vi "PID Straight Encoder.vi"(8 "error in":errorcluster, 10 "data":variant=variant(dbl -50.0), 11 "Auton Ref":T1={"queue"=refnum, "Drivetrain"={"DevStatus"={"status"=FALSE, "code"=0, "source"=""}, "Motors[]"=[{"DeviceStatus"={"status"=FALSE, "code"=0, "source"=""}, "Type"=enum."PWM", "PWM"={"PWM Channel"=enum."PWM 1", "DeadBand"={"Name"="SPARK", "maxPositivePwm"=1500, "minPositivePwm"=1010, "centerPwm"=1005, "maxNegativePwm"=1000, "minNegativePwm"=500, "angularRange"=0}}, "CAN"={"Device Number"=0, "SetOutput VI Ref"=variant(refnum<vi> refnum), "GetOutput VI Ref"=variant(refnum<vi> refnum), "Enable VI Ref"=variant(refnum<vi> refnum), "Disable VI Ref"=variant(refnum<vi> refnum), "Data"=variant}, "Invert"=TRUE}, {"DeviceStatus"={"status"=FALSE, "code"=0, "source"=""}, "Type"=enum."PWM", "PWM"={"PWM Channel"=enum."PWM 0", "DeadBand"={"Name"="SPARK", "maxPositivePwm"=1500, "minPositivePwm"=1010, "centerPwm"=1005, "maxNegativePwm"=1000, "minNegativePwm"=500, "angularRange"=0}}, "CAN"={"Device Number"=0, "SetOutput VI Ref"=variant(refnum<vi> refnum), "GetOutput VI Ref"=variant(refnum<vi> refnum), "Enable VI Ref"=variant(refnum<vi> refnum), "Disable VI Ref"=variant(refnum<vi> refnum), "Data"=variant}, "Invert"=FALSE}], "Square Inputs"=TRUE, "Max Output"=1.0}, "Encoder L"={"DevStatus"={"status"=FALSE, "code"=0, "source"=""}, "EncoderIndex"=enum."Enc 0", "CounterIndex"=enum."Invalid", "DistancePerCount"=0.0490874, "Decoding Type"=enum."4x"}, "Encoder R"={"DevStatus"={"status"=FALSE, "code"=0, "source"=""}, "EncoderIndex"=enum."Enc 1", "CounterIndex"=enum."Invalid", "DistancePerCount"=0.0490874, "Decoding Type"=enum."4x"}, "Gyro"={"DevStatus"={"status"=FALSE, "code"=0, "source"=""}, "Analog Channel"=enum."AI 1", "Offset"=0.0, "Gain (VoltsPerDegree/Second)"=0.0, "Gyro Type"=enum."XRS450", "Handle"=60, "SPI Bus"=enum."SPI On-Board, CS0", "Device Found"=TRUE, "Sample Rate"=1.0, "Calibrate On Open"=FALSE}, "Lock"={"notifier out"=refnum}, "Shifter"={"DevStatus"={"status"=FALSE, "code"=0, "source"=""}, "Pneumatics Control Module"=1, "Forward Solenoid Channel"=enum."Solenoid 0", "Reverse Solenoid Channel"=enum."Solenoid 1"}} {"Gyro"."Sample Rate" min=0.25 max=100.0 step=0.25}) -> (0 "error out":errorcluster)   [LabVIEW 2016, in "Drive System.lvlib"]
uses:
  Drive System.lvlib
  DriveMainType.ctl
  DriveCmd.ctl
  DriveCmdList.ctl
  <vilib>/Rock Robotics/WPI/RobotDrive/WPI_RobotDriveDevRef.ctl
  <vilib>/Rock Robotics/WPI/MotorControl/WPI_MotorControlDeviceRef.ctl
  <vilib>/Rock Robotics/WPI/MotorControl/WPI_MotorControlType.ctl
  <vilib>/Rock Robotics/SystemInterfaces/DIO/FPGA_DIOPWMChannel.ctl
  <vilib>/Rock Robotics/WPI/PWM/WPI_PWMDeadband.ctl
  <vilib>/Rock Robotics/WPI/Encoder/WPI_EncoderDevRef.ctl
  <vilib>/Rock Robotics/SystemInterfaces/Encoder/FPGA_EncoderIdx.ctl
  <vilib>/Rock Robotics/SystemInterfaces/Counter/FPGA_CounterCtrSystemIndex.ctl
  <vilib>/Rock Robotics/WPI/Encoder/WPI_EncoderType.ctl
  <vilib>/Rock Robotics/WPI/Gyro/WPI_GyroDevRef.ctl
  <vilib>/Rock Robotics/SystemInterfaces/AI/FPGA_AIChannel.ctl
  <vilib>/Rock Robotics/SystemInterfaces/spilib/spi_bus.ctl
  Varient Cmd Types/Lock Command.ctl
  <vilib>/Rock Robotics/WPI/Solenoid/WPI_SolenoidDevRef.ctl
  <vilib>/Rock Robotics/WPI/Solenoid/WPI_SolenoidChannel.ctl
  <vilib>/Platform/TimedLoop/XDataNode/timing_clust.ctl
  <vilib>/Platform/TimedLoop/XDataNode/nitl_modes.ctl
  <vilib>/Platform/TimedLoop/XDataNode/wakeup.ctl
  Varient Cmd Types/Drive PID CMD.ctl
  <vilib>/addons/control/pid/pid.llb/PID Output Rate Limiter (DBL).vi
  <vilib>/Platform/TimedLoop/XDataNode/XDataNode.xnode
  <vilib>/Platform/TimedLoop/XDataNode/XDNodeRunTimeDep.lvlib
  <vilib>/addons/control/pid/NI_PID_pid.lvlib
  <vilib>/ptbypt/NI_PtbyPt.lvlib
panel:
  in  "threshold":dbl=0.008
  out "mean":dbl=0.00016497888749945157 format="%0.2f"
  out "Waveform Chart 2":cluster{dbl, dbl}(graph)={-50.0, -50.00778875}
  out "Waveform Chart":dbl(graph)=0.02713616249999992
  in  "output range":cluster{"output high":dbl, "output low":dbl}={"output high"=1.0, "output low"=-1.0} {"output low" format="%.2f"; "output high" format="%.2f"}
  in  "i Zone":dbl=12.0 format="%.2f"
  in  "PIDF":cluster{"Kp":dbl, "Ki":dbl, "Kd":dbl, "Kf":dbl}={"Kp"=0.02, "Ki"=0.0, "Kd"=0.045, "Kf"=0.0} {"Kf" format="%.3f"; "Kd" format="%.3f"; "Ki" format="%.3f"; "Kp" format="%.3f"}
  in  "Gyro PIDF":cluster{"Kp":dbl, "Ki":dbl, "Kd":dbl, "Kf":dbl}={"Kp"=0.05, "Ki"=0.0, "Kd"=0.0, "Kf"=0.0} {"Kf" format="%.3f"; "Kd" format="%.3f"; "Ki" format="%.3f"; "Kp" format="%.3f"}
  in  "output rate":dbl=80.0 format="%.2f"
  # "Analog"
  # "XRS"
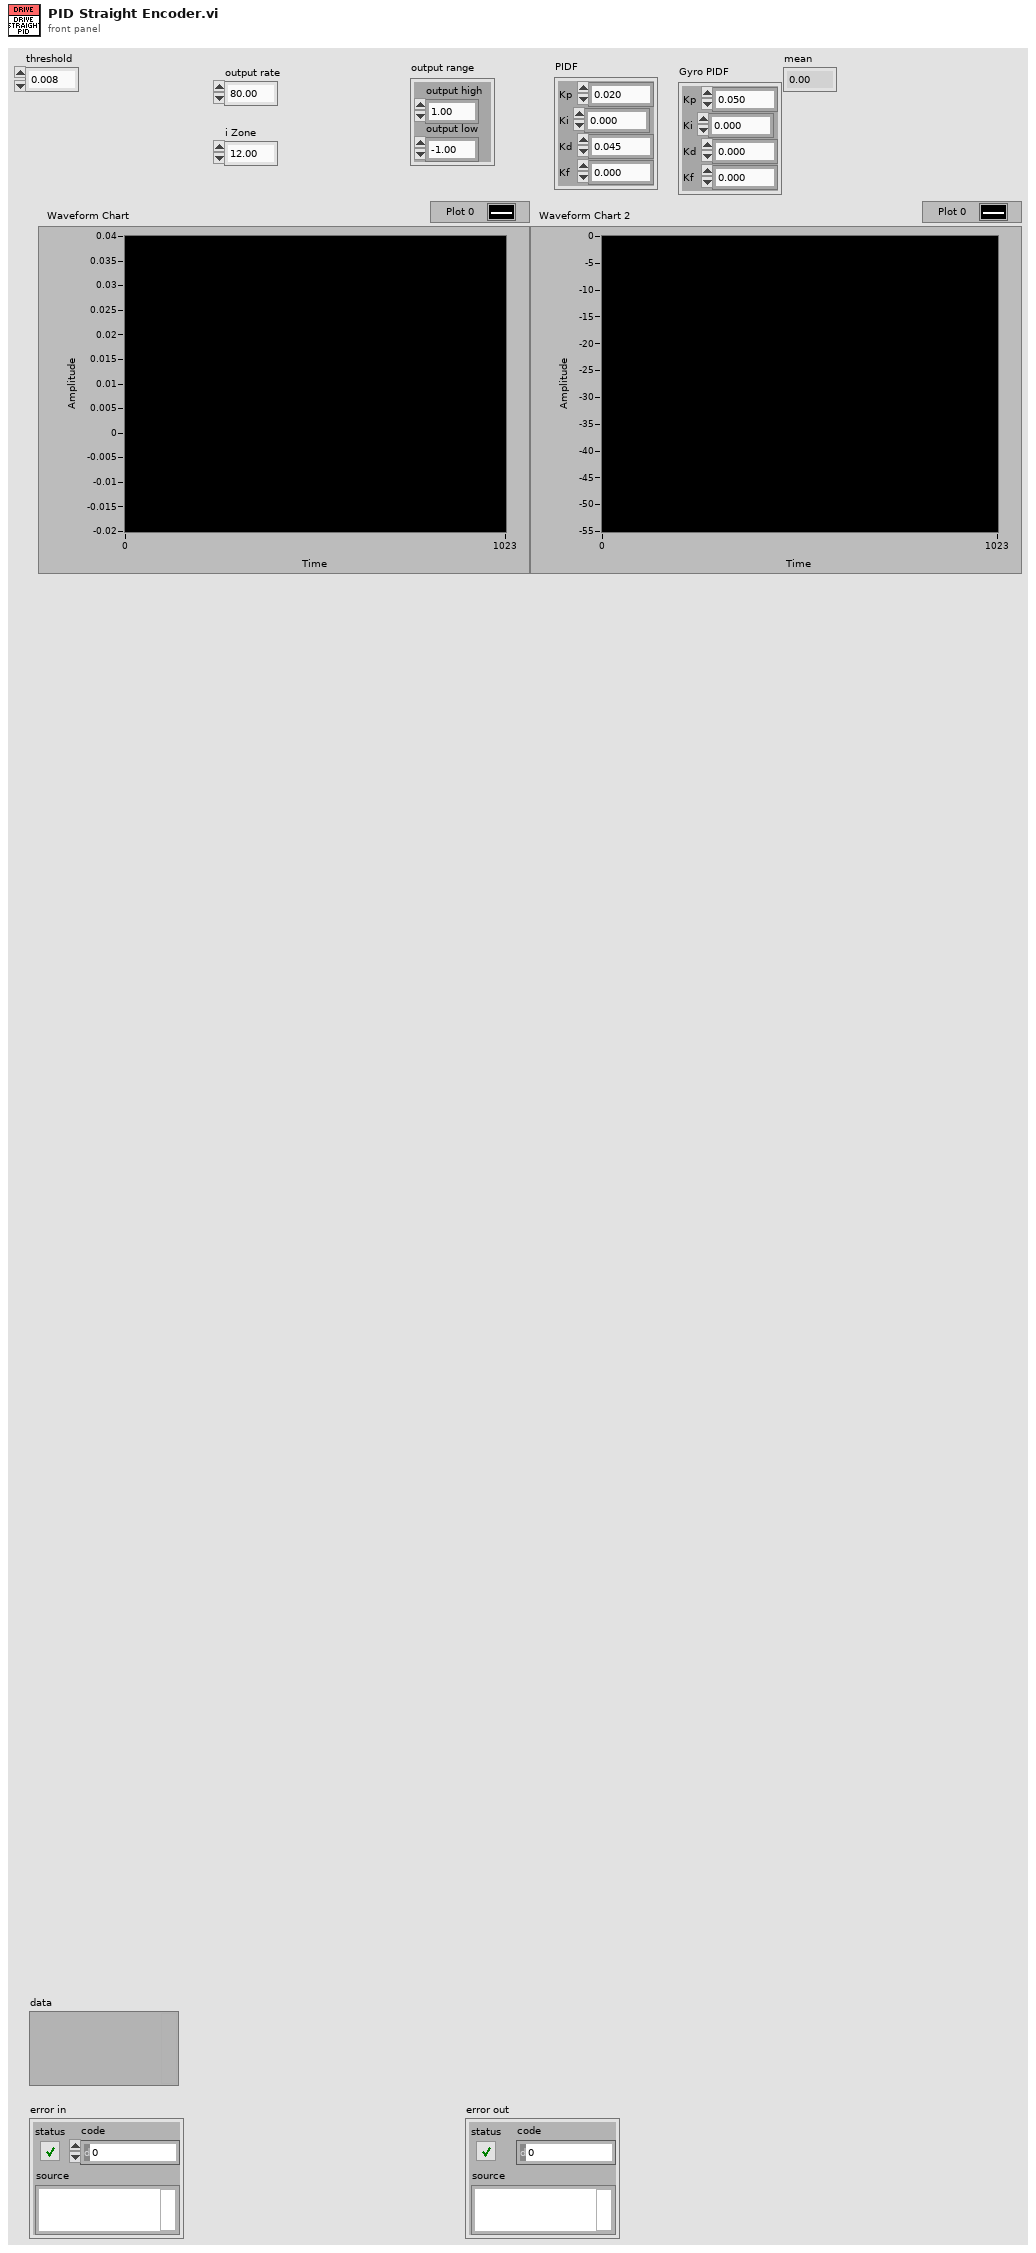
[diagram p1: front panel]
types:
  T1 = typedef "Drive System.lvlib/DriveMainType.ctl" = cluster{"queue":refnum<queue>, "Drivetrain":T2, "Encoder L":T7, "Encoder R":T7, "Gyro":T11, "Lock":T14, "Shifter":T15}
  T2 = typedef "WPI_RobotDriveDevRef.ctl" = cluster{"DevStatus":errorcluster, "Motors[]":T3[], "Square Inputs":bool, "Max Output":dbl}
  T3 = typedef "WPI_MotorControlDeviceRef.ctl" = cluster{"DeviceStatus":errorcluster, "Type":T4, "PWM":cluster{"PWM Channel":T5, "DeadBand":T6}, "CAN":cluster{"Device Number":u8, "SetOutput VI Ref":variant, "GetOutput VI Ref":variant, "Enable VI Ref":variant, "Disable VI Ref":variant, "Data":variant}, "Invert":bool}
  T4 = typedef "WPI_MotorControlType.ctl" = enum16{"PWM", "CAN"}
  T5 = typedef "FPGA_DIOPWMChannel.ctl" = enum8{"PWM 0", "PWM 1", "PWM 2", "PWM 3", "PWM 4", "PWM 5", "PWM 6", "PWM 7", "PWM 8", "PWM 9", "PWM MXP 0", "PWM MXP 1", "PWM MXP 2", "PWM MXP 3", "PWM MXP 4", "PWM MXP 5", "PWM MXP 6", "PWM MXP 7", "PWM MXP 8", "PWM MXP 9", "Invalid"}
  T6 = typedef "WPI_PWMDeadband.ctl" = cluster{"Name":string, "maxPositivePwm":i32, "minPositivePwm":i32, "centerPwm":i32, "maxNegativePwm":i32, "minNegativePwm":i32, "angularRange":u16}
  T7 = typedef "WPI_EncoderDevRef.ctl" = cluster{"DevStatus":errorcluster, "EncoderIndex":T8, "CounterIndex":T9, "DistancePerCount":dbl, "Decoding Type":T10}
  T8 = typedef "FPGA_EncoderIdx.ctl" = enum8{"Enc 0", "Enc 1", "Enc 2", "Enc 3", "Enc 4", "Enc 5", "Enc 6", "Enc 7", "Invalid"}
  T9 = typedef "FPGA_CounterCtrSystemIndex.ctl" = enum8{"Ctr 0", "Ctr 1", "Ctr 2", "Ctr 3", "Ctr 4", "Ctr 5", "Ctr 6", "Ctr 7", "Invalid"}
  T10 = typedef "WPI_EncoderType.ctl" = enum16{"1x", "2x", "4x"}
  T11 = typedef "WPI_GyroDevRef.ctl" = cluster{"DevStatus":errorcluster, "Analog Channel":T12, "Offset":dbl, "Gain (VoltsPerDegree/Second)":dbl, "Gyro Type":enum16{"Analog", "XRS450"}, "Handle":i32, "SPI Bus":T13, "Device Found":bool, "Sample Rate":dbl, "Calibrate On Open":bool}
  T12 = typedef "FPGA_AIChannel.ctl" = enum8{"AI 0", "AI 1", "AI 2", "AI 3", "AI MXP 0", "AI MXP 1", "AI MXP 2", "AI MXP 3", "Invalid"}
  T13 = typedef "spi_bus.ctl" = enum16{"SPI On-Board, CS0", "SPI On-Board, CS1", "SPI On-Board, CS2", "SPI On-Board, CS3", "SPI MXP", "Invalid"}
  T14 = typedef "Drive System.lvlib/Lock Command.ctl" = cluster{"notifier out":refnum<notifier>}
  T15 = typedef "WPI_SolenoidDevRef.ctl" = cluster{"DevStatus":errorcluster, "Pneumatics Control Module":u8, "Forward Solenoid Channel":T16, "Reverse Solenoid Channel":T16}
  T16 = typedef "WPI_SolenoidChannel.ctl" = enum8{"Solenoid 0", "Solenoid 1", "Solenoid 2", "Solenoid 3", "Solenoid 4", "Solenoid 5", "Solenoid 6", "Solenoid 7", "Invalid"}
  T17 = typedef "Drive System.lvlib/Drive PID CMD.ctl" = cluster{"distance":dbl, "angle offset (0)":dbl}
  T18 = typedef "XDNodeRunTimeDep.lvlib/timing_clust.ctl" = cluster{"Expected End [f-1]":u64, "Actual End [f-1]":u64, "Finished Late? [f-1]":bool, "Expected End [i-1]":u64, "Actual End [i-1]":u64, "Finished Late? [i-1]":bool, "Expected Start [i]":u64, "Actual Start [i]":u64, "Expected Start [f]":u64, "Actual Start [f]":u64, "Source Name":string, "Structure Name":string, "Period":i64, "Deadline":i64, "Offset":i64, "Start":i64, "Priority":i32, "Timeout":i32, "Mode":T19, "Wakeup Reason":T20, "Error":errorcluster, "Source Type":string, "Secondary Source Type":string, "Global End Time":u64, "Global Start Time":u64, "Frame Duration":u64, "Iteration Duration":u64, "Assigned CPU":i32, "I/O Scan Engine Mode":u32}
  T19 = typedef "XDNodeRunTimeDep.lvlib/nitl_modes.ctl" = enum32{"No Change", "Process missed periods, maintain original phase", "Discard missed periods, maintain original phase", "Process missed periods, ignore original phase", "Discard missed periods, ignore original phase"}
  T20 = typedef "XDNodeRunTimeDep.lvlib/wakeup.ctl" = enum32{"Normal", "Aborted", "Asynchronous wakeup", "Timing source error", "Timed loop error", "Timeout"}
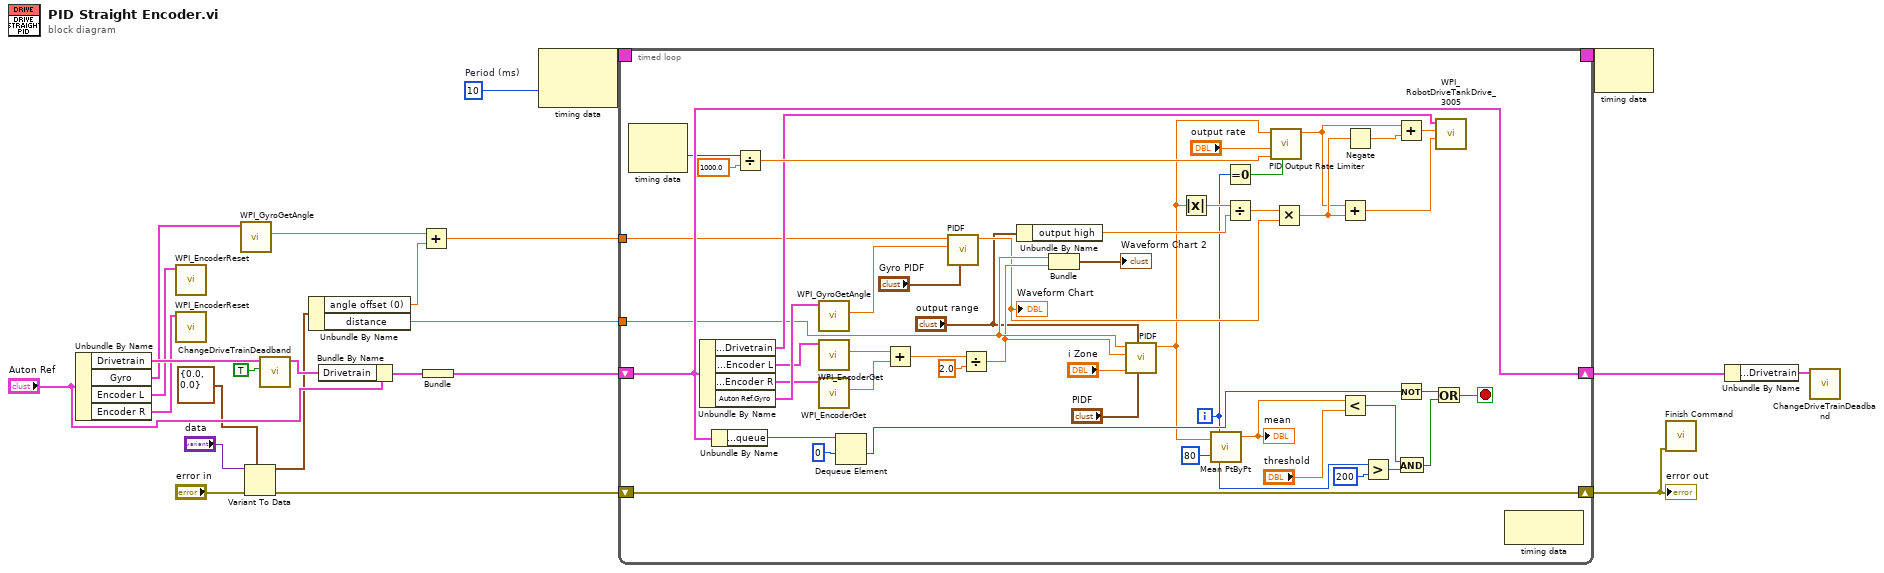
[diagram p0: block diagram]
diagram:
  w18 = i64 10  # Period (ms)
  n1 = Unbundle By Name("Auton Ref") -> ("Drivetrain"=w15:T2, "Gyro"=w10:T11, "Encoder L"=w8:T7, "Encoder R"=w7:T7)
  n2 = call <vilib>:"WPI_EncoderReset.vi"("EncoderDevRef"=w8) -> ()  [unwired: 9 in, 2 out]
  n3 = call <vilib>:"WPI_EncoderReset.vi"("EncoderDevRef"=w7) -> ()  [unwired: 9 in, 2 out]
  n4 = call <vilib>:"WPI_GyroGetAngle.vi"("GyroDevRef"=w10) -> ("Angle"=w9:dbl)  [unwired: 6 in, 4 out]
  n5 = Variant To Data(error in="error in", type=T17 {"distance"=0.0, "angle offset (0)"=0.0}, Variant="data") -> (data=w3:T17, error out=w22:errorcluster)
  n6 = call "ChangeDriveTrainDeadband.vi"("Eliminate Deadband"=TRUE, "Drivetrain in"=w15) -> ("Drivetrain out"=w13:T2)  [unwired: 9 in]
  n7 = Unbundle By Name(w3) -> ("angle offset (0)"=w2:dbl, "distance"=w1:dbl)
  n8 = Bundle By Name(cluster="Auton Ref", "Drivetrain"=w13) -> (w14:T1)
  n9 = Add(x=w9, y=w2) -> (x+y=w5:dbl)
  n10 = Bundle("Auton Ref"=w14) -> (w24:cluster{"Auton Ref":T1})  [unwired: 1 in]
  n11 = node-c288(w18) -> (w20:T18)  [unwired: 1 in]
  n12 = timed-loop {
    shift-right: [w69] -> w6
    shift-left: w22 -> [w69]
    shift-right: [w67] -> w12
    shift-left: w24 -> [w67]
    timing: w20 -> [_]
    timing-out: [_] -> w19
    tunnel: w5 -> [w53]
    tunnel: w1 -> [w47]
    i -> [w30]
    stop <- w36 stop-if-true
    n13 = node-c288() -> (w58:i64)  [unwired: 1 in, 1 out]
    n14 = Unbundle By Name(w67) -> ("Auton Ref.Drivetrain"=w55:T2, "Auton Ref.Encoder L"=w65:T7, "Auton Ref.Encoder R"=w64:T7, "Auton Ref.Gyro"=w66:T11)
    n15 = Unbundle By Name(w67) -> ("Auton Ref.queue"=w71:refnum<queue>)
    n16 = Divide(x=w58, y=1000.0) -> (x/y=w56:dbl)
    n17 = call <vilib>:"WPI_GyroGetAngle.vi"("GyroDevRef"=w66) -> ("Angle"=w54:dbl)  [unwired: 6 in, 4 out]
    n18 = call <vilib>:"WPI_EncoderGet.vi"("EncoderDevRef"=w65) -> ("Distance"=w63:dbl)  [unwired: 5 in, 5 out]
    n19 = call <vilib>:"WPI_EncoderGet.vi"("EncoderDevRef"=w64) -> ("Distance"=w62:dbl)  [unwired: 5 in, 5 out]
    n20 = Dequeue Element(queue=w71, timeout in ms (-1)=0) -> (timed out?=w70:bool)  [unwired: 1 in, 3 out]
    n21 = Add(x=w63, y=w62) -> (x+y=w61:dbl)
    n22 = call "PIDF.vi"("PIDF gains"="Gyro PIDF", "process variable"=w54, "setpoint"=w53) -> ("output"=w43:dbl)  [unwired: 6 in, 2 out]
    "Waveform Chart" <- w43
    n23 = Divide(x=w61, y=2.0) -> (x/y=w46:dbl)
    n24 = Unbundle By Name("output range") -> ("output high"=w38:dbl)
    n25 = Bundle("distance"=w47, w46) -> (→"Waveform Chart 2":cluster{"distance":dbl, dbl})  [unwired: 1 in]
    n26 = call "PIDF.vi"("PIDF gains"="PIDF", "output range"="output range", "i Zone"="i Zone", "process variable"=w46, "setpoint"=w47) -> ("output"=w25:dbl)  [unwired: 4 in, 2 out]
    n27 = Absolute Value(x=w25) -> (abs(x)=w40:dbl)
    n28 = call <vilib>:"Mean PtByPt.vi"("x"=w25, "sample length"=80) -> ("mean"=w33:dbl)  [unwired: 2 in, 1 out]
    "mean" <- w33
    n29 = Equal To 0?(x=w30) -> (x = 0?=w51:bool)
    n30 = Divide(x=w40, y=w38) -> (x/y=w37:dbl)
    n31 = call-poly <vilib>:"PID Output Rate Limiter.vi"("reinitialize? (F)"=w51, "dt (s)"=w56, "output rate (EGU/min)"="output rate", "input (controller output)"=w25) -> ("output"=w26:dbl)  [unwired: 4 in, 1 out]
    n32 = Multiply(x=w37, y=w43) -> (x*y=w41:dbl)
    n33 = Add(x=w26, y=w41) -> (x+y=w44:dbl)
    n34 = Less?(x=w33, y="threshold") -> (x < y?=w34:bool)
    n35 = Negate(x=w41) -> (-x=w42:dbl)
    n36 = Greater?(x=w30, y=200) -> (0:w28:bool)
    n37 = Add(x=w26, y=w42) -> (x+y=w45:dbl)
    n38 = Not(x=w70) -> (.not. x?=w48:bool)
    n39 = And(x=w34, y=w28) -> (x .and. y?=w31:bool)
    n40 = Or(x=w48, y=w31) -> (x .or. y?=w36:bool)
    n41 = call "WPI_RobotDriveTankDrive_3005.vi"("Right axis value"=w44, "Left axis value"=w45, "RobotDriveDevRef"=w55) -> ()  [unwired: 7 in, 2 out]
    n42 = node-c288() -> ()  [unwired: 1 in, 1 out]
  }
  "error out" <- w6
  n43 = node-c288(w19) -> ()  [unwired: 1 out]
  n44 = call "Finish Command.vi"("error in"=w6) -> ()  [unwired: 10 in, 1 out]
  n45 = Unbundle By Name(w12) -> ("Auton Ref.Drivetrain"=w11:T2)
  n46 = call "ChangeDriveTrainDeadband.vi"("Drivetrain in"=w11) -> ()  [unwired: 10 in, 1 out]
